vi "Set_Tunnel_Speed.vi"(3 "Mode":T1, 5 "Tunnel Velocity m/s":dbl min=0.0 max=50.0 format="%.2f") -> (0 "Error String":string)   [LabVIEW 2011]
doc: "This is an example of using features of the VI Server as a client. It shows how you might browse from one or more applications that may be exporting data from one or more data stations. \n\nThe example shows how to query a server for its list of exported VIs, how to get references to the VIs, and how call them with the Call By Reference function."
uses:
  Sub VIs/ADAM Controls/Tunnel_speed_mode.ctl
  Anemometry/Anemometry Sub Vis/File/Setup_Filetype.ctl
  Sub VIs/ADAM Controls/Channel_State.ctl
  Sub VIs/ADAM Controls/Calib_type_ADAM.ctl
  Sub VIs/ADAM Controls/Module_type_ADAM.ctl
  Sub VIs/ADAM Controls/Ch_description_ADAM.ctl
  Sub VIs/ADAM Controls/Function_ADAM.ctl
  Sub VIs/ADAM Controls/Address.ctl
  Anemometry/Anemometry Sub Vis/Controls/Global_mode.ctl
  Sub VIs/ADAM Controls/Update_scan_value.ctl
  Anemometry/Anemometry Sub Vis/Globals/Preference_global.vi
  Anemometry/Anemometry Sub Vis/Globals/Trav_pos_global.vi
  Anemometry/Anemometry Sub Vis/Globals/Constants_global.vi
  <vilib>/Analysis/NI_AALBase.lvlib
panel:
  in  "Set EnFlo Tun Speed":refnum<vi>
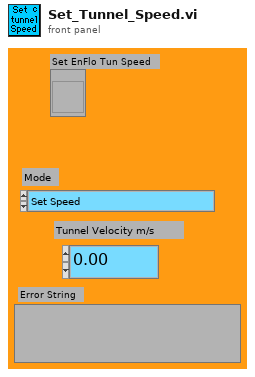
[diagram p1: front panel]
types:
  T1 = typedef "Tunnel_speed_mode.ctl" = enum16{"Set Speed", "Set Speed then wait", "Is tunnel speed allowable?"}
  T2 = typedef "Setup_Filetype.ctl" = enum16{"Measurement Setups", "Calibration Setups", "General", "Results File Plotter Setups", "Speed Calib Tweaks"}
  T3 = typedef "Channel_State.ctl" = enum16{"On", "Off", "Always On", "Always Off"}
  T4 = typedef "Calib_type_ADAM.ctl" = enum16{"Raw", "Bx + A", "Cx^2 + Bx + A", "Dx^3 + Cx^2 + Bx + A", "In Band", "Hi-Tec Q", "Hi-Tec M_dot", "Text"}
  T5 = typedef "Module_type_ADAM.ctl" = enum16{"4011", "4012", "4013", "4014", "4016", "4017", "4018", "4021", "4050", "4052", "4053", "4060", "4080", "5000", "5017", "5018", "5024", "5051", "5056", "5060", "6060", "Tracker", "WEST", "GILL", "JEM", "VICI", "Vaisala", "DRUCK", "Run VI Named:", "IR2100", "PPT", "Comparator", "VIRTUAL", "Hold Value", "Read A", "Read Ch", "Coded", "Client Info", "Web Client", "X10", "Test"}
  T6 = typedef "Ch_description_ADAM.ctl" = cluster{"Ch Name":string, "Type":T5, "Function":T7, "Ch State":T3, "Calibration type":T4, "A":dbl, "B":dbl, "C":dbl, "D":dbl, "Comments":string, "Address":T8, "String":string, "Duty":u16}
  T7 = typedef "Function_ADAM.ctl" = enum16{"Analogue Input", "Digital Input", "Event counter", "Event rate", "Analogue Output", "Digital Output", "Relay Output"}
  T8 = typedef "Address.ctl" = cluster{"Main":i32, "Ch.":i32, "Sub":i32, "Port Name":string}
  T9 = typedef "Global_mode.ctl" = enum16{"Read Global", "Load Global From File", "Write Global to File"}
  T10 = typedef "Update_scan_value.ctl" = cluster{"Channel Name":string, "New Value":dbl}
  T11 = typedef "Server_Comms.ctl" = enum16{"Server Link Healthy", "Do Not Link To Server"}
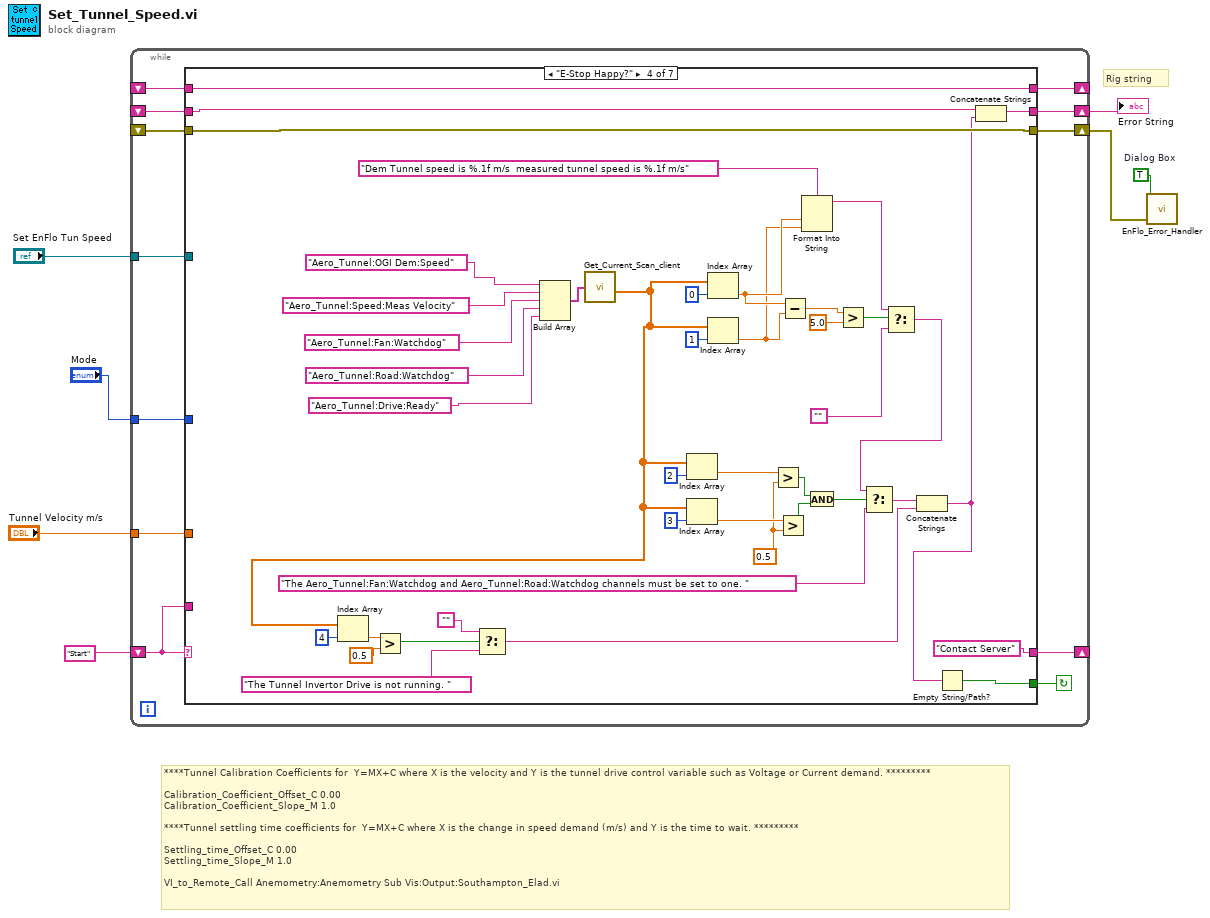
[diagram p0: block diagram]
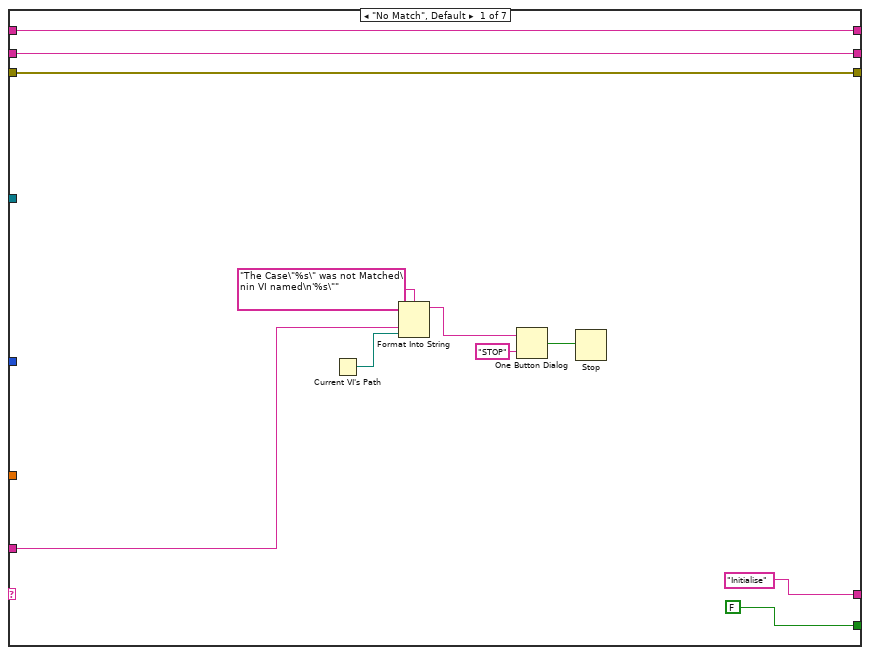
[diagram p2: hidden frame]
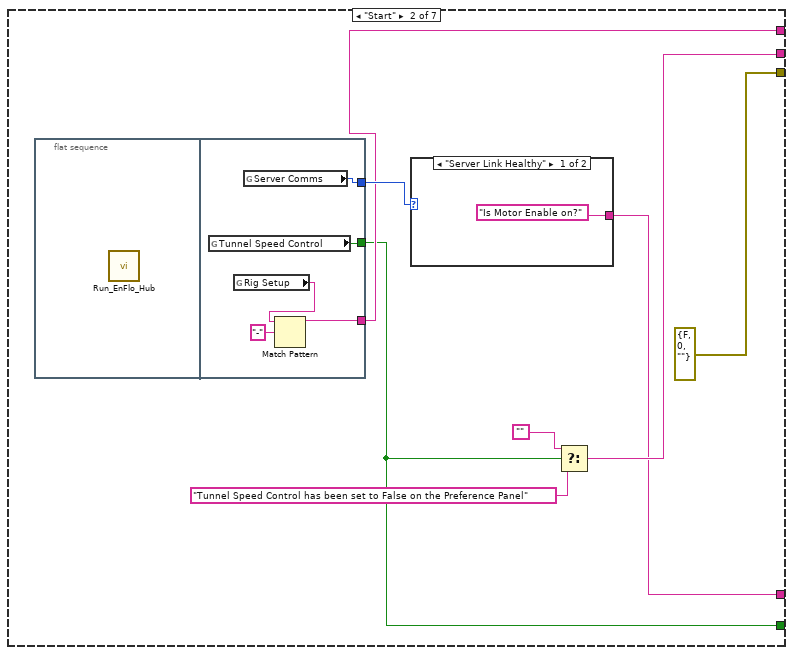
[diagram p3: hidden frame]
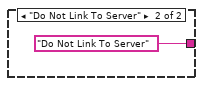
[diagram p4: hidden frame]
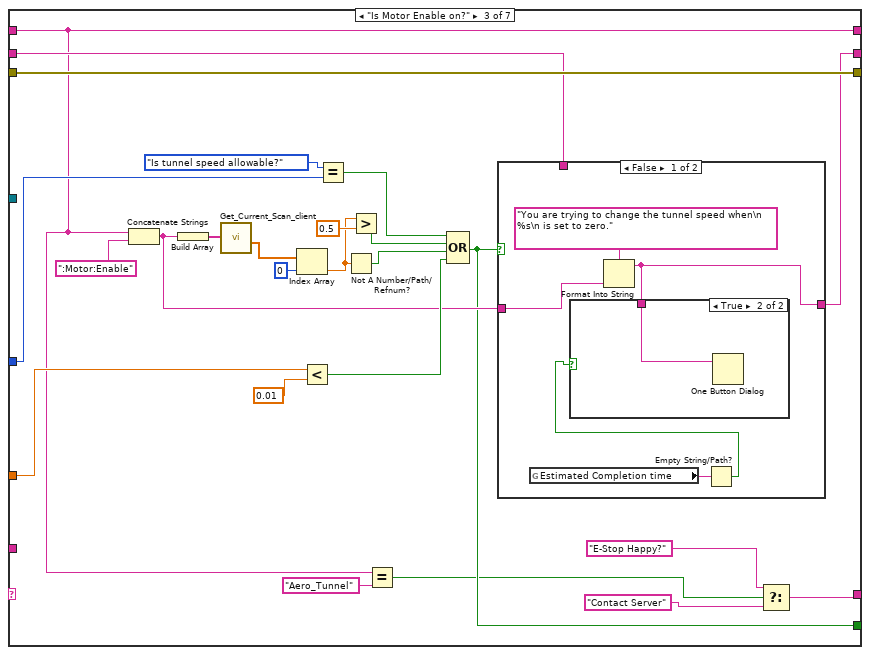
[diagram p5: hidden frame]
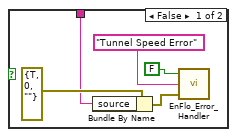
[diagram p6: hidden frame]
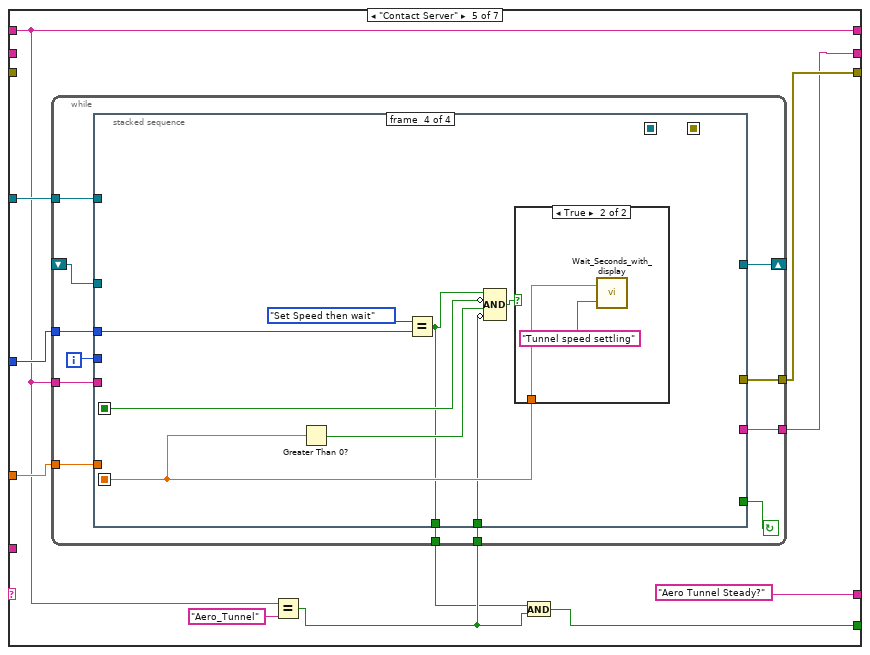
[diagram p8: hidden frame]
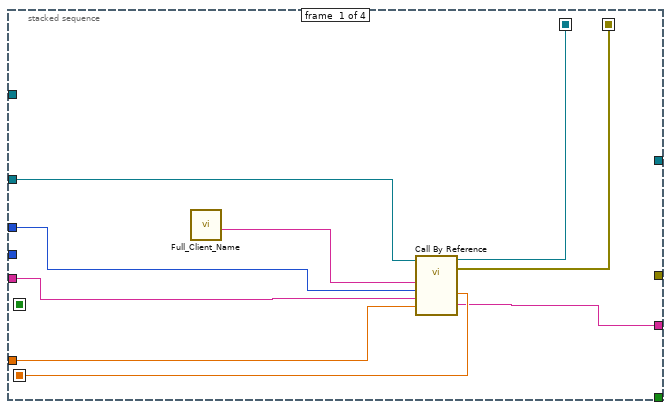
[diagram p9: hidden frame]
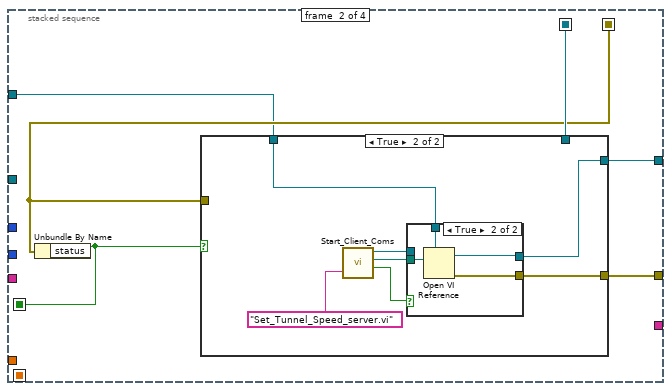
[diagram p10: hidden frame]
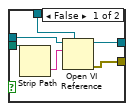
[diagram p12: hidden frame]
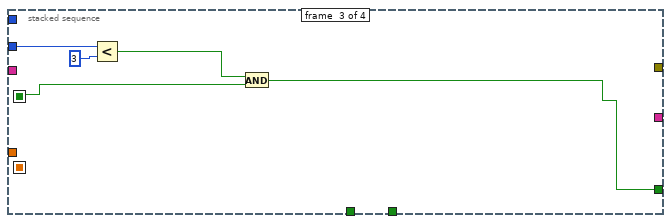
[diagram p13: hidden frame]
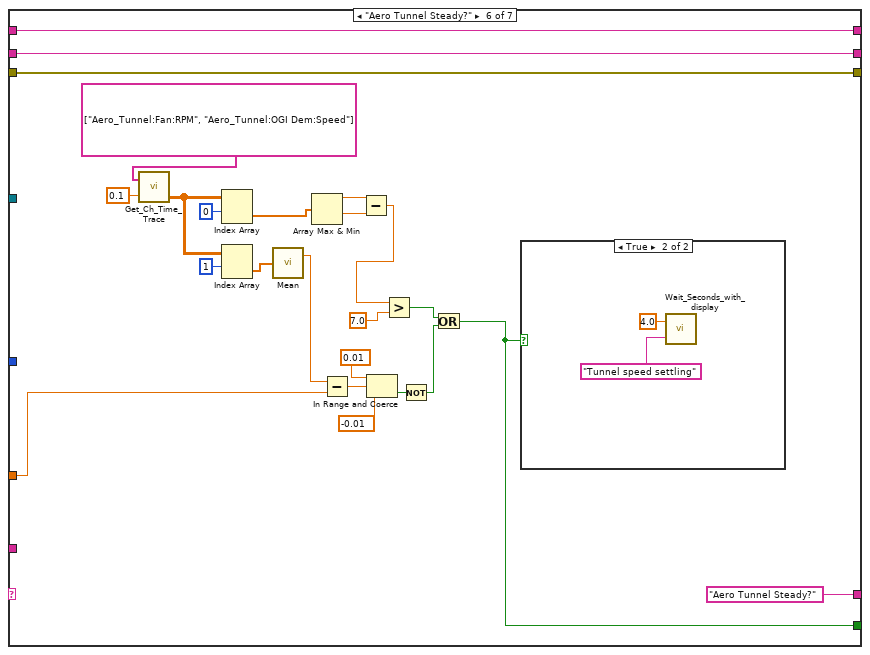
[diagram p15: hidden frame]
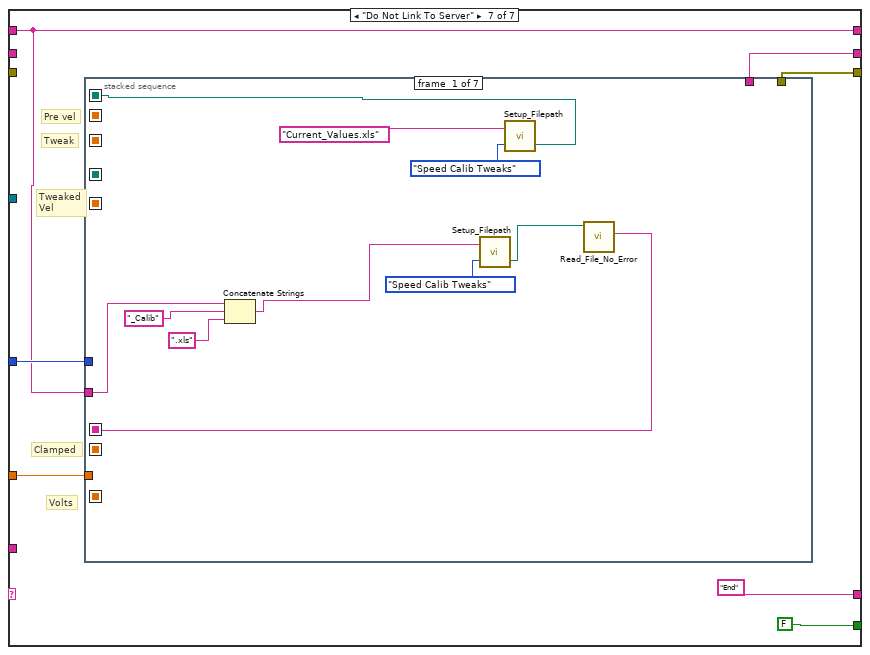
[diagram p17: hidden frame]
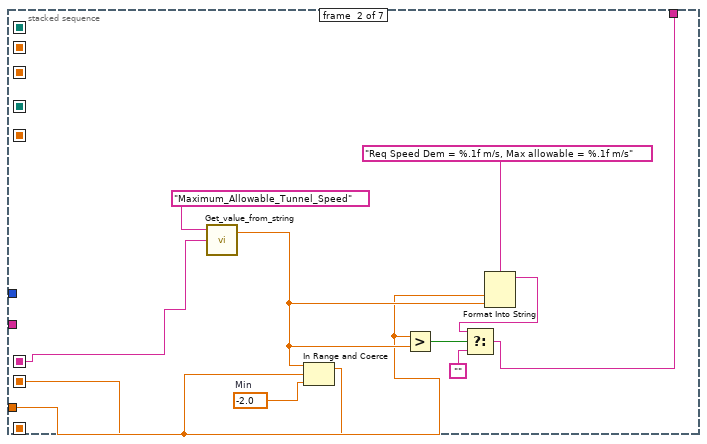
[diagram p18: hidden frame]
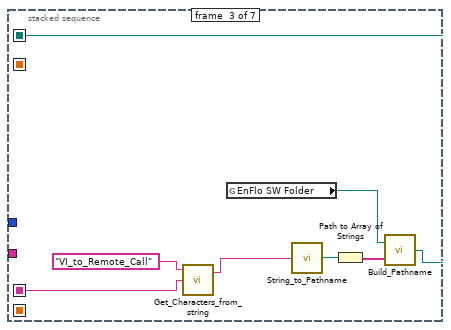
[diagram p19: hidden frame]
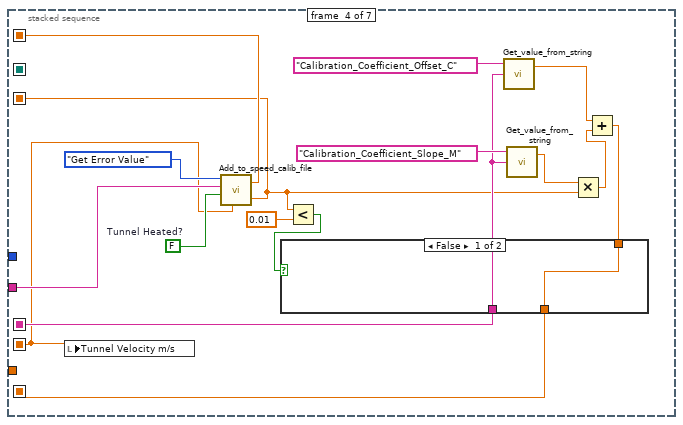
[diagram p20: hidden frame]
diagram:
  w7 = TRUE  # Dialog Box
  # "Rig string"
  # "****Tunnel Calibration Coefficients for  Y=MX+C where X is the velocity and Y is the tunnel drive control variable such as Voltage or Current demand. *********\n\nCalibration_Coefficient_Offset_C\t0.00\nCalibration_Coefficient_Slope_M\t1.0\n\n****Tunnel settling time coefficients for  Y=MX+C where X is the change in speed demand (m/s) and Y is the time to wait. *********\n\nSettling_time_Offset_C\t0.00\nSettling_time_Slope_M\t1.0\n\nVI_to_Remote_Call\tAnemometry:Anemometry Sub Vis:Output:Southampton_Elad.vi"
  n1 = while {
    shift-left: "Start" -> [w18]
    shift-right: [w19] -> _
    shift-right: [w17] -> w5
    shift-left: _ -> [w16]
    shift-right: [w15] -> w4
    shift-left: _ -> [w10]
    tunnel: "Mode" -> [w14]
    tunnel: "Tunnel Velocity m/s" -> [w13]
    shift-right: [w12] -> _
    shift-left: _ -> [w11]
    tunnel: "Set EnFlo Tun Speed" -> [w8]
    stop <- w9 continue-if-true
    n2 = case shown="\"E-Stop Happy?\"" w18 {
      tunnel: [FALSE w35 w55 w94 w125 w202 FALSE] -> w9
      tunnel: ["Initialise" w31 w47 "Contact Server" ("f") "Aero Tunnel Steady?" ("f") "Aero Tunnel Steady?" ("f") "End"] -> w19
      tunnel: w18 -> [w25 _ _ _ _ _ _]
      tunnel: [w22 w33 w57 w115 w132 w218 w225] -> w17
      tunnel: w16 -> [w22 _ w56 w116 _ w218 _]
      tunnel: [w20 errorcluster {"status"=FALSE, "code"=0, "source"=""} ("error out") w59 w110 w133 w217 w224] -> w15
      tunnel: w14 -> [_ _ w53 _ w135 _ w227]
      tunnel: w13 -> [_ _ w60 _ w134 w209 w226]
      tunnel: [w21 w36 w50 w124 w129 w219 w223] -> w12
      tunnel: w11 -> [w21 _ w50 w124 w129 w219 w223]
      tunnel: w10 -> [w20 _ w59 w110 _ w217 _]
      tunnel: w8 -> [_ _ _ _ w131 _ _]
      frame "No Match", Default {
        n3 = Current VI's Path() -> (path=w24:path)
        n4 = Format Into String(format string="The Case\"%s\" was not Matched\nin VI named\n'%s\"" ("Format String"), w25, w24) -> (resulting string=w28:string)  [unwired: 2 in, 1 out]
        n5 = One Button Dialog(message=w28, button name ("OK")="STOP") -> (true=w26:bool)
        n6 = Stop(stop? (T)=w26) -> ()
      }
      frame "Start" {
        n7 = flat-sequence {
          tunnel: [w45] -> w38
          tunnel: [w44] -> w35
          tunnel: [w41] -> w36
          frame #0 {
            n8 = call "Run_EnFlo_Hub.vi"() -> ()  [unwired: 8 out]
          }
          frame #1 {
            n9 = global read "Preference_global.vi" "Tunnel Speed Control"() -> (w44:bool)
            n10 = global read "Preference_global.vi" "Rig Setup"() -> (w43:string)
            n11 = global read "Preference_global.vi" "Server Comms"() -> (w45:T11)
            n12 = Match Pattern(string=w43, regular expression="-") -> (before substring=w41:string)  [unwired: 4 out]
          }
        }
        n13 = case shown="\"Server Link Healthy\"" w38 {
          tunnel: ["Is Motor Enable on?" "Do Not Link To Server"] -> w31
          frame "Server Link Healthy" {
          }
          frame "Do Not Link To Server" {
          }
        }
        n14 = Select(t="", s=w35, f="Tunnel Speed Control has been set to False on the Preference Panel" ("Error String")) -> (s? t:f=w33:string)
      }
      frame "Is Motor Enable on?" {
        n15 = Concatenate Strings(w50, ":Motor:Enable" ("string")) -> (w58:string)
        n16 = Build Array(w58) -> (w62:string[])
        n17 = call "Get_Current_Scan_client.vi"("ADAM Ch Names"=w62) -> ("Numerical Values"=w63:dbl[])  [unwired: 3 out]
        n18 = Index Array(array=w63, index=0) -> (element=w65:dbl)
        n19 = Less?(x=w60, y=0.01) -> (x < y?=w70:bool)
        n20 = Equal?(x=Tunnel_speed_mode."Is tunnel speed allowable?" ("Mode"), y=w53) -> (x = y?=w52:bool)
        n21 = Not A Number/Path/Refnum?(number/path/refnum=w65) -> (NaN/Path/Refnum?=w67:bool)
        n22 = Greater?(x=w65, y=0.5) -> (0:w68:bool)
        n23 = Equal?(x=w50, y="Aero_Tunnel") -> (x = y?=w49:bool)
        n24 = Compound Arithmetic op=OR(w52, w68, w67, w70) -> (w55:bool)
        n25 = case shown="False" w55 {
          tunnel: w58 -> [w74 _]
          tunnel: [w71 w82] -> w57
          tunnel: w56 -> [_ w82]
          frame False {
            n26 = global read "Trav_pos_global.vi" "Estimated Completion time"() -> (w73:string)
            n27 = Format Into String(format string="You are trying to change the tunnel speed when\n %s\n is set to zero.", w74) -> (resulting string=w71:string)  [unwired: 2 in, 1 out]
            n28 = Empty String/Path?(string/path=w73) -> (empty?=w72:bool)
            n29 = case shown="True" w72 {
              tunnel: w71 -> [w77 w81]
              frame False {
                n30 = Bundle By Name(cluster=errorcluster {"status"=TRUE, "code"=0, "source"=""} ("error in (no error)"), "source"=w77) -> (w78:errorcluster)
                n31 = call "EnFlo_Error_Handler.vi"("error in (no error)"=w78, "Error Type"="Tunnel Speed Error", "Dialog Box (T)"=FALSE) -> ()  [unwired: 3 out]
              }
              frame True {
                n32 = One Button Dialog(message=w81) -> ()  [unwired: 2 out]
              }
            }
          }
          frame True {
          }
        }
        n33 = Select(t="E-Stop Happy?" ("f"), s=w49, f="Contact Server") -> (s? t:f=w47:string)
      }
      frame "E-Stop Happy?" {
        w101 = 0.5 ("y")
        n34 = Build Array("Aero_Tunnel:OGI Dem:Speed", "Aero_Tunnel:Speed:Meas Velocity", "Aero_Tunnel:Fan:Watchdog", "Aero_Tunnel:Road:Watchdog", "Aero_Tunnel:Drive:Ready") -> (w121:string[])
        n35 = call "Get_Current_Scan_client.vi"("ADAM Ch Names"=w121) -> ("Numerical Values"=w91:dbl[])  [unwired: 1 in, 2 out]
        n36 = Index Array(array=w91, index=4) -> (element=w90:dbl)
        n37 = Greater?(x=w90, y=0.5) -> (0:w88:bool)
        n38 = Select(t="", s=w88, f="The Tunnel Invertor Drive is not running. ") -> (s? t:f=w84:string)
        n39 = Index Array(array=w91, index=2) -> (element=w103:dbl)
        n40 = Index Array(array=w91, index=3) -> (element=w102:dbl)
        n41 = Index Array(array=w91, index=0) -> (element=w114:dbl)
        n42 = Index Array(array=w91, index=1) -> (element=w113:dbl)
        n43 = Greater?(x=w103, y=w101) -> (0:w99:bool)
        n44 = Greater?(x=w102, y=w101) -> (0:w100:bool)
        n45 = Subtract(x=w114, y=w113) -> (x-y=w118:dbl)
        n46 = Format Into String(format string="Dem Tunnel speed is %.1f m/s  measured tunnel speed is %.1f m/s", w114, w113) -> (resulting string=w111:string)  [unwired: 2 in, 1 out]
        n47 = And(x=w99, y=w100) -> (x .and. y?=w96:bool)
        n48 = Greater?(x=w118, y=5.0) -> (0:w108:bool)
        n49 = Select(t=w111, s=w108, f="") -> (s? t:f=w97:string)
        n50 = Select(t=w97, s=w96, f="The Aero_Tunnel:Fan:Watchdog and Aero_Tunnel:Road:Watchdog channels must be set to one. ") -> (s? t:f=w85:string)
        n51 = Concatenate Strings(w85, w84) -> (w83:string)
        n52 = Empty String/Path?(string/path=w83) -> (empty?=w94:bool)
        n53 = Concatenate Strings(w116, w83) -> (w115:string)
      }
      frame "Contact Server" {
        n54 = Equal?(x=w129, y="Aero_Tunnel") -> (x = y?=w127:bool)
        n55 = while {
          tunnel: w135 -> [w142]
          tunnel: w134 -> [w143]
          tunnel: [w144] -> w133
          shift-left: _ -> [w139]
          shift-right: [w147] -> _
          tunnel: [w141] -> w132
          tunnel: w129 -> [w140]
          tunnel: w131 -> [w138]
          tunnel: w127 -> [w137]
          tunnel: [w136] -> w126
          i -> [w146]
          stop <- w145 continue-if-true
          n56 = stacked-sequence {
            seq-local: [w155 _ _ _] -> [_ w161 _ _]
            seq-local: [w154 _ _ _] -> [_ w159 _ _]
            seq-local: [_ w160 _ _] -> [_ _ w183 w190]
            seq-local: [w151 _ _ _] -> [_ _ _ w193]
            tunnel: w139 -> [w156 _ _ _]
            tunnel: [_ w162 _ _] -> w147
            tunnel: w146 -> [_ _ w184 _]
            tunnel: [_ _ w182 _] -> w145
            tunnel: [_ w158 _ _] -> w144
            tunnel: w143 -> [w152 _ _ _]
            tunnel: w142 -> [w148 _ _ w194]
            tunnel: [w150 _ _ _] -> w141
            tunnel: w140 -> [w149 _ _ _]
            tunnel: w138 -> [_ w157 _ _]
            tunnel: w137 -> [_ _ _ w188]
            tunnel: [_ _ _ w187] -> w136
            frame #0 {
              n57 = call "Full_Client_Name.vi"() -> ("Client Name"=w153:string)
              n58 = call-by-ref "?"(reference=w156, "Tunnel Velocity m/s"=w152, "Rig Name"=w149, "Mode"=w148, "Client Name"=w153) -> (reference out=w155:refnum<vi>, error out=w154:errorcluster, "Error String"=w150:string, "Settling Time (s)"=w151:dbl)  [unwired: 1 in, 1 out]
            }
            frame #1 {
              n59 = Unbundle By Name(w159) -> ("status"=w160:bool)
              n60 = case shown="True" w160 {
                tunnel: [w163 w167] -> w162
                tunnel: w161 -> [w163 _]
                tunnel: [w164 w166] -> w158
                tunnel: w159 -> [w164 _]
                tunnel: w157 -> [_ w165]
                frame False {
                }
                frame True {
                  n61 = call "Start_Client_Coms.vi"("VI name to run on server"="Set_Tunnel_Speed_server.vi") -> ("LabVIEW application reference"=w169:refnum<vi>, "Checked VI name"=w170:path, "Local Call"=w168:bool)  [unwired: 1 in, 1 out]
                  n62 = case shown="True" w168 {
                    tunnel: [w176 w181] -> w167
                    tunnel: w165 -> [w174 w180]
                    tunnel: w170 -> [w173 w179]
                    tunnel: w169 -> [w172 _]
                    tunnel: [w175 w178] -> w166
                    frame False {
                      n63 = Strip Path(path=w173) -> (name=w177:string)  [unwired: 1 out]
                      n64 = Open VI Reference(type specifier VI Refnum (for type only)=w174, application reference (local)=w172, vi path=w177) -> (vi reference=w176:refnum<vi>, error out=w175:errorcluster)  [unwired: 1 in, 2 out]
                    }
                    frame True {
                      n65 = Open VI Reference(type specifier VI Refnum (for type only)=w180, vi path=w179) -> (vi reference=w181:refnum<vi>, error out=w178:errorcluster)  [unwired: 1 in, 3 out]
                    }
                  }
                }
              }
            }
            frame #2 {
              n66 = Less?(x=w184, y=3) -> (x < y?=w186:bool)
              n67 = And(x=w186, y=w183) -> (x .and. y?=w182:bool)
            }
            frame #3 {
              n68 = Greater Than 0?(x=w193) -> (x > 0?=w189:bool)
              n69 = Equal?(x=Tunnel_speed_mode."Set Speed then wait" ("Mode"), y=w194) -> (x = y?=w187:bool)
              n70 = Compound Arithmetic op=AND(w187, invert w190, w189, invert w188) -> (w191:bool)
              n71 = case shown="True" w191 {
                tunnel: w193 -> [_ w195]
                frame False {
                }
                frame True {
                  n72 = call "Wait_Seconds_with_display.vi"("Message"="Tunnel speed settling", "Seconds to wait"=w195) -> ()  [unwired: 2 out]
                }
              }
            }
          }
        }
        n73 = And(x=w126, y=w127) -> (x .and. y?=w125:bool)
      }
      frame "Aero Tunnel Steady?" {
        n74 = call "Get_Ch_Time_Trace.vi"("Desired Ch Names"=string[] ["Aero_Tunnel:Fan:RPM", "Aero_Tunnel:OGI Dem:Speed"] ("ADAM Ch Names"), "History Length (mins)"=0.1) -> ("Output array"=w212:dbl[][])  [unwired: 2 out]
        n75 = Index Array(array=w212, index (row)=0) -> (element=w208:dbl[])  [unwired: 1 in]
        n76 = Index Array(array=w212, index (row)=1) -> (element=w211:dbl[])  [unwired: 1 in]
        n77 = call <vilib>:"Mean.vi"("X"=w211) -> ("mean"=w210:dbl)  [unwired: 1 out]
        n78 = Array Max & Min(array=w208) -> (max value=w207:dbl, min value=w206:dbl)  [unwired: 2 out]
        n79 = Subtract(x=w210, y=w209) -> (x-y=w199:dbl)
        n80 = Subtract(x=w207, y=w206) -> (x-y=w205:dbl)
        n81 = In Range and Coerce(upper limit=0.01, x=w199, lower limit=-0.01) -> (In Range?=w198:bool)  [unwired: 1 out]
        n82 = Greater?(x=w205, y=7.0) -> (0:w203:bool)
        n83 = Not(x=w198) -> (.not. x?=w197:bool)
        n84 = Or(x=w203, y=w197) -> (x .or. y?=w202:bool)
        n85 = case shown="True" w202 {
          frame False {
          }
          frame True {
            n86 = call "Wait_Seconds_with_display.vi"("Message"="Tunnel speed settling", "Seconds to wait"=4.0) -> ()  [unwired: 2 out]
          }
        }
      }
      frame "Do Not Link To Server" {
        # "Clamped"
        # "Pre vel"
        # "Tweak"
        # "Tweaked\nVel"
        # "Volts"
        n87 = stacked-sequence {
          seq-local: [w236 _ _ _ _ _ _] -> [_ w250 w256 w264 w280 w339 _]
          seq-local: [_ _ w251 _ _ _ _] -> [_ _ _ _ w284 _ _]
          seq-local: [_ _ _ w260 _ _ _] -> [_ _ _ _ w279 _ w352]
          seq-local: [_ _ _ w263 _ _ _] -> [_ _ _ _ w282 w334 _]
          seq-local: [_ _ _ _ w281 _ _] -> [_ _ _ _ _ w333 _]
          seq-local: [_ _ _ w265 _ _ _] -> [_ _ _ _ _ _ w358]
          seq-local: [w233 _ _ _ _ _ _] -> [_ _ _ _ _ _ w360]
          seq-local: [_ w241 _ _ _ _ _] -> [_ _ _ w258 _ _ w357]
          tunnel: w226 -> [_ w242 _ _ _ _ _]
          tunnel: w223 -> [w237 _ _ w273 _ _ w354]
          tunnel: w227 -> [_ _ _ _ w283 w328 _]
          tunnel: [_ w240 _ _ _ _ _] -> w225
          tunnel: [_ _ _ _ w278 _ _] -> w224
          frame #0 {
            n88 = Concatenate Strings(w237, "_Calib" ("Substring"), ".xls" ("string")) -> (w231:string)
            n89 = call "Setup_Filepath.vi"("Setup File Type"=Setup_Filetype."Speed Calib Tweaks", "Filename in"=w231) -> ("Filename Out"=w230:path)  [unwired: 1 out]
            n90 = call "Setup_Filepath.vi"("Setup File Type"=Setup_Filetype."Speed Calib Tweaks", "Filename in"="Current_Values.xls" ("name or relative path")) -> ("Filename Out"=w233:path)  [unwired: 1 out]
            n91 = call "Read_File_No_Error.vi"("Filename"=w230) -> ("string"=w236:string)  [unwired: 2 in, 7 out]
          }
          frame #1 {
            w244 = -2.0  # Min
            n92 = call "Get_value_from_string.vi"("Input string"=w250, "Variable name"="Maximum_Allowable_Tunnel_Speed") -> ("Value"=w243:dbl)  [unwired: 1 in, 1 out]
            n93 = In Range and Coerce(upper limit=w243, x=w242, lower limit=w244) -> (coerced(x)=w241:dbl)  [unwired: 1 out]
            n94 = Greater?(x=w242, y=w243) -> (0:w245:bool)
            n95 = Format Into String(format string="Req Speed Dem = %.1f m/s, Max allowable = %.1f m/s", w242, w243) -> (resulting string=w247:string)  [unwired: 2 in, 1 out]
            n96 = Select(t=w247, s=w245, f="") -> (s? t:f=w240:string)
          }
          frame #2 {
            n97 = call "Get_Characters_from_string.vi"("Input string"=w256, "Variable name"="VI_to_Remote_Call") -> ("Value"=w254:string)  [unwired: 1 in, 1 out]
            n98 = global read "Constants_global.vi" "EnFlo SW Folder"() -> (w252:path)
            n99 = call "String_to_Pathname.vi"("Input String"=w254) -> ("path"=w255:path)
            n100 = Path to Array of Strings(0:w255) -> (2:w253:string[])  [unwired: 1 out]
            n101 = call "Build_Pathname.vi"("Output Array"=w253, "Pathname"=w252) -> ("Appended path"=w251:path)
          }
          frame #3 {
            w271 = FALSE  # Tunnel Heated?
            n102 = local write "Tunnel Velocity m/s"(w258) -> ()
            n103 = call "Add_to_speed_calib_file.vi"("Desired Velocity"=w258, "Tunnel Heated?"=w271, "Rig Name"=w273, "Mode"=enum16{"Add Row", "Get Error Value"}."Get Error Value") -> ("Tweaked Demand"=w263:dbl, "Calib Tweak %"=w265:dbl)  [unwired: 2 in]
            n104 = Less?(x=w263, y=0.01) -> (x < y?=w261:bool)
            n105 = call "Get_value_from_string.vi"("Input string"=w264, "Variable name"="Calibration_Coefficient_Offset_C") -> ("Value"=w266:dbl)  [unwired: 1 in, 1 out]
            n106 = call "Get_value_from_string.vi"("Input string"=w264, "Variable name"="Calibration_Coefficient_Slope_M") -> ("Value"=w268:dbl)  [unwired: 1 in, 1 out]
            n107 = Multiply(x=w268, y=w263) -> (x*y=w267:dbl)
            n108 = Add(x=w266, y=w267) -> (x+y=w259:dbl)
            n109 = case shown="False" w261 {
              tunnel: w264 -> [_ w276]
              tunnel: [w274 w275] -> w260
              tunnel: w259 -> [w274 _]
              frame False {
              }
              frame True {
                n110 = call "Get_value_from_string.vi"("Input string"=w276, "Variable name"="Zero_Velocity_Output_Voltage") -> ("Value"=w275:dbl)  [unwired: 1 in, 1 out]
              }
            }
          }
          frame #4 {
            n111 = while {
              tunnel: w284 -> [w294]
              tunnel: w283 -> [w293]
              tunnel: w282 -> [w292]
              tunnel: [w291] -> w281
              shift-right: [w289] -> _
              shift-left: _ -> [w288]
              tunnel: [w287] -> w278
              tunnel: w280 -> [w286]
              tunnel: w279 -> [w285]
              stop <- TRUE stop-if-true
              n112 = case shown="\"Set Speed then wait\", Default" w293 {
                tunnel: w294 -> [_ w314]
                tunnel: w292 -> [_ w301]
                tunnel: [w296 w303] -> w291
                tunnel: [w296 w301] -> w289
                tunnel: w288 -> [w296 w302]
                tunnel: [errorcluster {"status"=FALSE, "code"=0, "source"=""} ("error out") w297] -> w287
                tunnel: w286 -> [_ _]
                tunnel: w285 -> [_ w300]
                frame "Is tunnel speed allowable?" {
                }
                frame "Set Speed then wait", Default {
                  n113 = Open VI Reference(type specifier VI Refnum (for type only)=refnum<vi> refnum, vi path=w314) -> (vi reference=w312:refnum<vi>, error out=w311:errorcluster)  [unwired: 1 in, 3 out]
                  n114 = property class="VI Interface Type 0"(reference=w312, error in=w311) -> (reference out=w309:refnum<vi>, error out=w310:errorcluster, "Front Panel.Open"=w308:bool)
                  n115 = case shown="False" w308 {
                    tunnel: w310 -> [w319 w322]
                    tunnel: w309 -> [w318 w323]
                    tunnel: [w317 w323] -> w307
                    tunnel: [w316 w322] -> w306
                    tunnel: [0.0 ("Tweaked Demand") w321] -> w303
                    tunnel: w302 -> [_ w321]
                    frame False {
                      n116 = property class="VI Interface Type 0"(reference=w318, error in=w319, "Front Panel.Open"=TRUE ("Front Panel Window:Open")) -> (reference out=w317:refnum<vi>, error out=w316:errorcluster)
                    }
                    frame True {
                    }
                  }
                  n117 = call-by-ref "?"(reference=w307, error in=w306, "Demand"=w300) -> (reference out=w304:refnum<vi>, error out=w305:errorcluster, "error out"=w298:errorcluster)
                  n118 = Close Reference(reference=w304, error in (no error)=w305) -> (error out=w299:errorcluster)
                  n119 = Select(t=w299, s=w299, f=w298) -> (s? t:f=w297:errorcluster)
                }
              }
            }
          }
          frame #5 {
            n120 = Subtract(x=w333, y=w334) -> (x-y=w332:dbl)
            n121 = Absolute Value(x=w332) -> (abs(x)=w326:dbl)
            n122 = call "Get_value_from_string.vi"("Input string"=w339, "Variable name"="Settling_time_Offset_C") -> ("Value"=w335:dbl)  [unwired: 1 in, 1 out]
            n123 = call "Get_value_from_string.vi"("Input string"=w339, "Variable name"="Settling_time_Slope_M") -> ("Value"=w337:dbl)  [unwired: 1 in, 1 out]
            n124 = Multiply(x=w337, y=w326) -> (x*y=w336:dbl)
            n125 = Add(x=w335, y=w336) -> (x+y=w327:dbl)
            n126 = Greater?(x=w326, y=0.05) -> (0:w324:bool)
            n127 = Equal?(x=Tunnel_speed_mode."Set Speed then wait" ("Mode"), y=w328) -> (x = y?=w330:bool)
            n128 = Compound Arithmetic op=AND(w324, w330) -> (w329:bool)
            n129 = case shown="False" w329 {
              tunnel: w327 -> [_ w341]
              frame False {
              }
              frame True {
                n130 = call "Wait_Seconds_with_display.vi"("Message"="Tunnel speed settling", "Seconds to wait"=w341) -> ()  [unwired: 2 out]
              }
            }
          }
          frame #6 {
            n131 = Concatenate Strings(w354, ":Speed:Dem_Voltage" ("string")) -> (w349:string)
            n132 = Bundle By Name(cluster=T10 {"Channel Name"="", "New Value"=0.0} ("Update Scan Value Cluster"), "Channel Name"=w349, "New Value"=w352) -> (w355:T10)
            n133 = call "Value_to_string.vi"("Value"=w358, "Label for value"="Calib Tweak") -> ("Output string"=w363:string)  [unwired: 1 in]
            n134 = call "Value_to_string.vi"("Value"=w357, "Label for value"="Velocity Demand") -> ("Output string"=w362:string)  [unwired: 1 in]
            n135 = Concatenate Strings(w363, w362) -> (w361:string)
            n136 = Bundle By Name(cluster=T6 {"Ch Name"="", "Type"=enum."4011", "Function"=enum."Analogue Input", "Ch State"=enum."On", "Calibration type"=enum."Raw", "A"=0.0, "B"=0.0, "C"=0.0, "D"=0.0, "Comments"="", "Address"={"Main"=0, "Ch."=0, "Sub"=0, "Port Name"=""}, "String"="", "Duty"=0} ("Ch Discription"), "Ch Name"=w349, "Type"=Module_type_ADAM."Hold Value", "Calibration type"=Calib_type_ADAM."Raw", "Ch State"=Channel_State."On") -> (w343:T6)
            n137 = call "Write_File_Simple.vi"("append to file? (new file:F)"=FALSE, "character string"=w361, "file path"=w360) -> ()  [unwired: 2 out]
            n138 = Build Array(w355) -> (w345:T10[])
            n139 = Build Array(w343) -> (w344:T6[])
            n140 = call "Read_Write_Local_table.vi"("Mode"=Global_mode."Write Global to File", "Ch Values in"=w345, "Channels Descriptions In"=w344) -> ()  [unwired: 3 out]
          }
        }
      }
    }
  }
  "Error String" <- w5
  n141 = call "EnFlo_Error_Handler.vi"("error in (no error)"=w4, "Dialog Box (T)"=w7) -> ()  [unwired: 1 in, 3 out]
